vi "Write output cluster.vi"(8 "error in (no error)":errorcluster, 9 "output cluster":T1, 11 "S4GUI in":refnum<class "S4GUI.lvclass">) -> (0 "error out":errorcluster, 3 "S4GUI out":refnum<class "S4GUI.lvclass">)   [LabVIEW 2018, in "S4GUI.lvclass"]
uses:
  S4GUI.lvclass
  S4GUI.lvclass/S4GUI.ctl
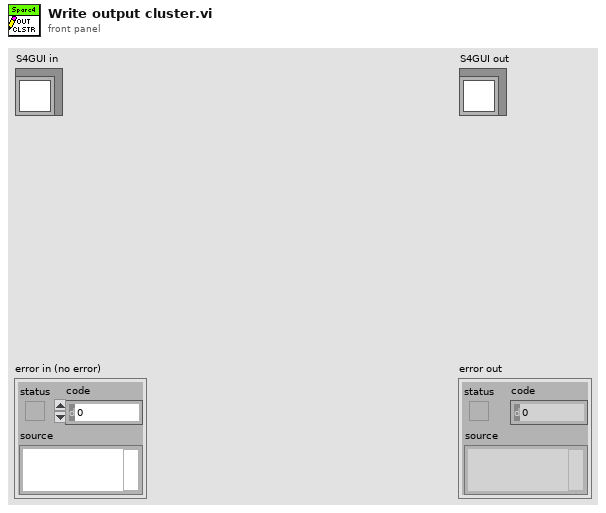
[diagram p1: front panel]
types:
  T1 = cluster{"Trigger Mode Status":string, "String output":string, "Instrument Status":cluster{"WPROT pos":dbl, "WPSEL pos":dbl, "GMIR pos":dbl, "GFOC pos":dbl, "CALW pos":dbl, "ASEL pos":dbl, "mode":bool, "String Status":string, "connection":bool, "operational":bool}, "Sync Box State":i32, "Trigger General Status":string, "Instrument States":cluster{"WPSEL State":i32, "WPROT State":i32, "CALW State":i32, "ASEL State":i32, "GMIR State":i32, "GFOC State":i32}, "Instrument Pos Names":cluster{"WPROT posname":string, "WPSEL posname":string, "CALW posname":string, "ASEL posname":string}, "ChannelA_Status":cluster{"Current exp":dbl, "Frames done":u32, "LastFileImage":string, "CamStatus":string, "Run state":u32, "connection":bool, "Cooler ON/OFF":i16, "Currently temperature":i16, "Temperature Status":string, "target  temp":i16, "conf runing":bool, "FT":bool, "UsedDisk":u16, "operational":bool}, "WPROT seq":u16, "ChannelB_Status":cluster{"Current exp":dbl, "Frames done":u32, "LastFileImage":string, "CamStatus":string, "Run state":u32, "connection":bool, "Cooler ON/OFF":i16, "Currently temperature":i16, "Temperature Status":string, "target  temp":i16, "conf runing":bool, "FT":bool, "UsedDisk":u16, "operational":bool}, "ChannelC_Status":cluster{"Current exp":dbl, "Frames done":u32, "LastFileImage":string, "CamStatus":string, "Run state":u32, "connection":bool, "Cooler ON/OFF":i16, "Currently temperature":i16, "Temperature Status":string, "target  temp":i16, "conf runing":bool, "FT":bool, "UsedDisk":u16, "operational":bool}, "ChannelD_Status":cluster{"Current exp":dbl, "Frames done":u32, "LastFileImage":string, "CamStatus":string, "Run state":u32, "connection":bool, "Cooler ON/OFF":i16, "Currently temperature":i16, "Temperature Status":string, "target  temp":i16, "conf runing":bool, "FT":bool, "UsedDisk":u16, "operational":bool}, "ChannelA_CCD":cluster{"ACQUISITION_MODE":u8, "TRIGGER_MODE":u8, "READ_MODE":u8, "PREAMP":u8, "READOUT_RATE":u8, "VERTICAL_SHIFT_SPEED":u8, "EM_MODE":u8, "EM_GAIN":u16, "SHUTTER_MODE":u8, "SHUTTER_TTL":u8, "SHUTTER_OPENNING_TIME":u16, "SHUTTER_CLOSING_TIME":u16, "VBIN":u16, "HBIN":u16, "INITIAL_LINE":u16, "INITIAL_COLUMN":u16, "FINAL_LINE":u16, "FINAL_COLUMN":u16, "FRAME_TRANSFER":bool, "VERTICAL_CLOCK_VOLTAGE":u8, "AD_CHANNEL":u32}, "ChannelB_CCD ":cluster{"ACQUISITION_MODE":u8, "TRIGGER_MODE":u8, "READ_MODE":u8, "PREAMP":u8, "READOUT_RATE":u8, "VERTICAL_SHIFT_SPEED":u8, "EM_MODE":u8, "EM_GAIN":u16, "SHUTTER_MODE":u8, "SHUTTER_TTL":u8, "SHUTTER_OPENNING_TIME":u16, "SHUTTER_CLOSING_TIME":u16, "VBIN":u16, "HBIN":u16, "INITIAL_LINE":u16, "INITIAL_COLUMN":u16, "FINAL_LINE":u16, "FINAL_COLUMN":u16, "FRAME_TRANSFER":bool, "VERTICAL_CLOCK_VOLTAGE":u8, "AD_CHANNEL":u32}, "ChannelC_CCD":cluster{"ACQUISITION_MODE":u8, "TRIGGER_MODE":u8, "READ_MODE":u8, "PREAMP":u8, "READOUT_RATE":u8, "VERTICAL_SHIFT_SPEED":u8, "EM_MODE":u8, "EM_GAIN":u16, "SHUTTER_MODE":u8, "SHUTTER_TTL":u8, "SHUTTER_OPENNING_TIME":u16, "SHUTTER_CLOSING_TIME":u16, "VBIN":u16, "HBIN":u16, "INITIAL_LINE":u16, "INITIAL_COLUMN":u16, "FINAL_LINE":u16, "FINAL_COLUMN":u16, "FRAME_TRANSFER":bool, "VERTICAL_CLOCK_VOLTAGE":u8, "AD_CHANNEL":u32}, "ChannelD_CCD":cluster{"ACQUISITION_MODE":u8, "TRIGGER_MODE":u8, "READ_MODE":u8, "PREAMP":u8, "READOUT_RATE":u8, "VERTICAL_SHIFT_SPEED":u8, "EM_MODE":u8, "EM_GAIN":u16, "SHUTTER_MODE":u8, "SHUTTER_TTL":u8, "SHUTTER_OPENNING_TIME":u16, "SHUTTER_CLOSING_TIME":u16, "VBIN":u16, "HBIN":u16, "INITIAL_LINE":u16, "INITIAL_COLUMN":u16, "FINAL_LINE":u16, "FINAL_COLUMN":u16, "FRAME_TRANSFER":bool, "VERTICAL_CLOCK_VOLTAGE":u8, "AD_CHANNEL":u32}, "CHA_Checked Params":cluster{"ACQUISITION_MODE":bool, "TRIGGER_MODE":bool, "READ_MODE":bool, "PREAMP":bool, "READOUT_RATE":bool, "VERTICAL_SHIFT_SPEED":bool, "EM_MODE":bool, "EM_GAIN":bool, "SHUTTER_MODE":bool, "SHUTTER_TTL":bool, "SHUTTER_OPENING_TIME":bool, "SHUTTER_CLOSING_TIME":bool, "VBIN":bool, "HBIN":bool, "INITIAL_LINE":bool, "INITIAL_COLUMN":bool, "FINAL_LINE":bool, "FINAL_COLUMN":bool, "FRAME_TRANSFER":bool, "VERTICAL_CLOCK_VOLTAGE":bool, "AD_CHANNEL":bool}, "CHB_Checked Params":cluster{"ACQUISITION_MODE":bool, "TRIGGER_MODE":bool, "READ_MODE":bool, "PREAMP":bool, "READOUT_RATE":bool, "VERTICAL_SHIFT_SPEED":bool, "EM_MODE":bool, "EM_GAIN":bool, "SHUTTER_MODE":bool, "SHUTTER_TTL":bool, "SHUTTER_OPENING_TIME":bool, "SHUTTER_CLOSING_TIME":bool, "VBIN":bool, "HBIN":bool, "INITIAL_LINE":bool, "INITIAL_COLUMN":bool, "FINAL_LINE":bool, "FINAL_COLUMN":bool, "FRAME_TRANSFER":bool, "VERTICAL_CLOCK_VOLTAGE":bool, "AD_CHANNEL":bool}, "CHC_Checked Params":cluster{"ACQUISITION_MODE":bool, "TRIGGER_MODE":bool, "READ_MODE":bool, "PREAMP":bool, "READOUT_RATE":bool, "VERTICAL_SHIFT_SPEED":bool, "EM_MODE":bool, "EM_GAIN":bool, "SHUTTER_MODE":bool, "SHUTTER_TTL":bool, "SHUTTER_OPENING_TIME":bool, "SHUTTER_CLOSING_TIME":bool, "VBIN":bool, "HBIN":bool, "INITIAL_LINE":bool, "INITIAL_COLUMN":bool, "FINAL_LINE":bool, "FINAL_COLUMN":bool, "FRAME_TRANSFER":bool, "VERTICAL_CLOCK_VOLTAGE":bool, "AD_CHANNEL":bool}, "CHD_Checked Params":cluster{"ACQUISITION_MODE":bool, "TRIGGER_MODE":bool, "READ_MODE":bool, "PREAMP":bool, "READOUT_RATE":bool, "VERTICAL_SHIFT_SPEED":bool, "EM_MODE":bool, "EM_GAIN":bool, "SHUTTER_MODE":bool, "SHUTTER_TTL":bool, "SHUTTER_OPENING_TIME":bool, "SHUTTER_CLOSING_TIME":bool, "VBIN":bool, "HBIN":bool, "INITIAL_LINE":bool, "INITIAL_COLUMN":bool, "FINAL_LINE":bool, "FINAL_COLUMN":bool, "FRAME_TRANSFER":bool, "VERTICAL_CLOCK_VOLTAGE":bool, "AD_CHANNEL":bool}, "Trigger_connection":bool, "TCSPD_connection":bool, "TCS extended":string, "TCS id":u32, "S4ICS id":u32, "focus pos":i32, "Focus_connection":bool, "WS_connection":bool, "weather status":cluster{"broker":string, "version":string, "date":string, "hour":string, "outHumidity":string, "inHumidity":string, "inTemp":string, "outTemp":string, "windSpeed":string, "windDirection":string, "pressure":string, "dewOut":string, "dewIn":string, "leaf":string, "rain":string, "windChill":string}, "GS STATUS cluster":cluster{"FocusPhot":dbl, "FocusPolar":dbl, "FocusEffic":dbl, "FocusInstrum":dbl, "ICS":bool, "AG":bool, "BROKER":string}, "TCSPD_operational":bool, "Focus_operational":bool, "object_suffix":string, "dflat_suffix":string, "sflat_suffix":string, "dark_suffix":string, "zero_suffix":string, "focus_suffix":string, "suffixAlertVisible":bool}
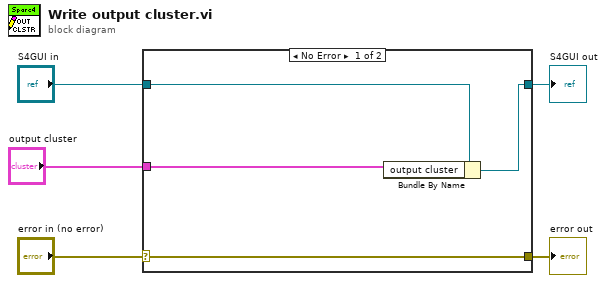
[diagram p0: block diagram]
diagram:
  n1 = case shown="No Error" "error in (no error)" {
    selector: "error in (no error)" -> [w9 w10]
    tunnel: [w9 w10] -> w4
    tunnel: [w7 w11] -> w2
    tunnel: "S4GUI in" -> [w8 w11]
    tunnel: "output cluster" -> [w6 _]
    frame No Error {
      n2 = Bundle By Name(cluster=w8, "output cluster"=w6) -> (w7:refnum<class "S4GUI.lvclass">)
    }
    frame Error {
    }
  }
  "error out" <- w4
  "S4GUI out" <- w2
